vi "Aim Camera.vi"(6 "Target Y":dbl, 7 "Target X":dbl, 8 "time difference (ms)":i16, 9 "Old Y":dbl, 11 "Old X":dbl) -> (0 "Y In Range?":bool, 1 "Current Y":dbl, 2 "X In Range?":bool, 3 "Current X":dbl)   [LabVIEW 2013]
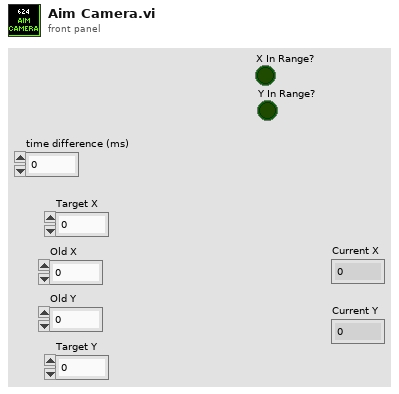
[diagram p1: front panel]
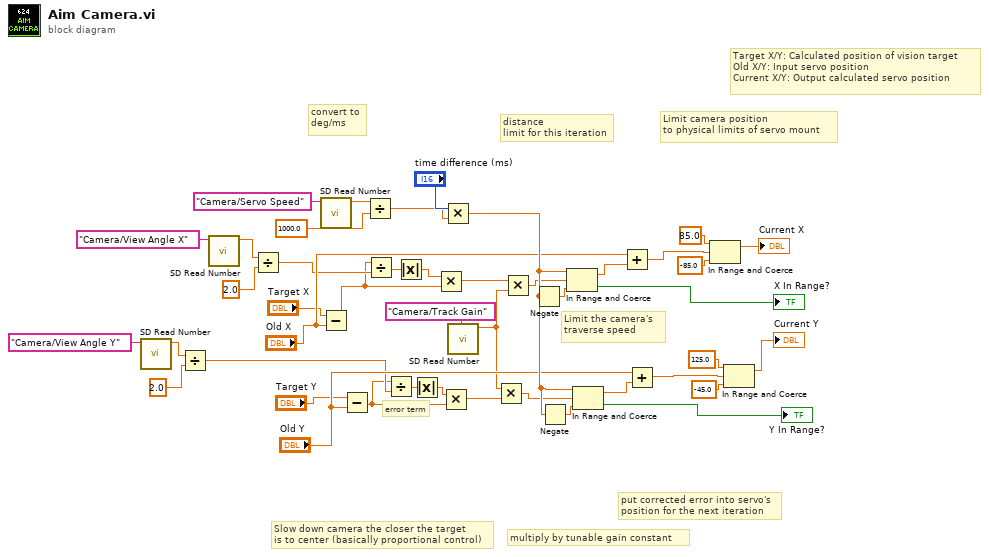
[diagram p0: block diagram]
diagram:
  # "put corrected error into servo's\nposition for the next iteration"
  # "error term"
  # "Limit camera position \nto physical limits of servo mount"
  # "multiply by tunable gain constant"
  # "Slow down camera the closer the target \nis to center (basically proportional control)"
  # "Limit the camera's \ntraverse speed"
  # "Target X/Y: Calculated position of vision target\nOld X/Y: Input servo position\nCurrent X/Y: Output calculated servo position"
  # "distance\nlimit for this iteration"
  # "convert to\ndeg/ms"
  n1 = call <vilib>:"SD Read Number.vi"("Name"="Camera/View Angle Y") -> ("Numeric"=w15:dbl)  [unwired: 8 in, 2 out]
  n2 = Divide(x=w15, y=2.0) -> (x/y=w13:dbl)
  n3 = call <vilib>:"SD Read Number.vi"("Name"="Camera/View Angle X") -> ("Numeric"=w21:dbl)  [unwired: 8 in, 2 out]
  n4 = Divide(x=w21, y=2.0) -> (x/y=w18:dbl)
  n5 = call <vilib>:"SD Read Number.vi"("Name"="Camera/Servo Speed") -> ("Numeric"=w43:dbl)  [unwired: 8 in, 2 out]
  n6 = Subtract(x="Target X", y="Old X") -> (x-y=w6:dbl)
  n7 = Subtract(x="Target Y", y="Old Y") -> (x-y=w5:dbl)
  n8 = Divide(x=w43, y=1000.0) -> (x/y=w40:dbl)
  n9 = Divide(x=w6, y=w18) -> (x/y=w3:dbl)
  n10 = Divide(x=w5, y=w13) -> (x/y=w1:dbl)
  n11 = Absolute Value(x=w3) -> (abs(x)=w4:dbl)
  n12 = Absolute Value(x=w1) -> (abs(x)=w2:dbl)
  n13 = Multiply(x=w4, y=w6) -> (x*y=w10:dbl)
  n14 = Multiply(x=w2, y=w5) -> (x*y=w8:dbl)
  n15 = Multiply(x="time difference (ms)", y=w40) -> (x*y=w37:dbl)
  n16 = call <vilib>:"SD Read Number.vi"("Name"="Camera/Track Gain") -> ("Numeric"=w7:dbl)  [unwired: 8 in, 2 out]
  n17 = Multiply(x=w7, y=w8) -> (x*y=w9:dbl)
  n18 = Multiply(x=w10, y=w7) -> (x*y=w11:dbl)
  n19 = Negate(x=w37) -> (-x=w39:dbl)
  n20 = Negate(x=w37) -> (-x=w38:dbl)
  n21 = In Range and Coerce(upper limit=w37, x=w11, lower limit=w39) -> (coerced(x)=w34:dbl, In Range?=→"X In Range?":bool)
  n22 = In Range and Coerce(upper limit=w37, x=w9, lower limit=w38) -> (coerced(x)=w32:dbl, In Range?=→"Y In Range?":bool)
  n23 = Add(x="Old X", y=w34) -> (x+y=w27:dbl)
  n24 = Add(x="Old Y", y=w32) -> (x+y=w23:dbl)
  n25 = In Range and Coerce(upper limit=85.0, x=w27, lower limit=-85.0) -> (coerced(x)=→"Current X":dbl)  [unwired: 1 out]
  n26 = In Range and Coerce(upper limit=125.0, x=w23, lower limit=-45.0) -> (coerced(x)=→"Current Y":dbl)  [unwired: 1 out]
